vi "Get RD Data.vi"(8 "error in":errorcluster, 11 "tCRD in":refnum<class "tCRD.lvclass">) -> (0 "error out":errorcluster, 3 "tCRD out":refnum<class "tCRD.lvclass">)   [LabVIEW 2015, in "tCRD.lvclass"]
uses:
  tCRD.lvclass
  tCRD.lvclass/tCRD.ctl
  Reusable/Instrument/Instrument.lvclass/Instrument.ctl
  Reusable/CRDS/Main/CRDS.lvclass/CRDS.ctl
  Accessors/Read FPGA Ref.vi
  Accessors/Read RepRate.vi
  Accessors/Read SamplesPerRep.vi
  Reusable/Instrument/Write Restart Requested_.vi
  Reusable/CRDS/Main/Write Laser Data.vi
  <vilib>/Utility/error.llb/Error Cluster From Error Code.vi
  <vilib>/rvi/errors/niLvFpgaAdjustHostInterfaceError.vi
  tFPGA Ref.ctl
  <vilib>/rvi/interface/nirviMethod/nirviMethod.xnode
  FPGA Bitfiles/Handix_OpenPathCRD.lvbitx
  <vilib>/FPGAPlugInAG/sbRIO-9637/niLvFpga_ReadFifo_sbRIO-9637.vi
  <vilib>/rvi/errors/niLvFpgaMergeErrorWithErrorCode.vi
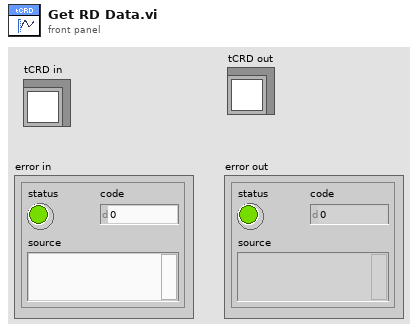
[diagram p1: front panel]
types:
  T1 = typedef "tCRD.lvclass/tFPGA Ref.ctl" = refnum<k20>
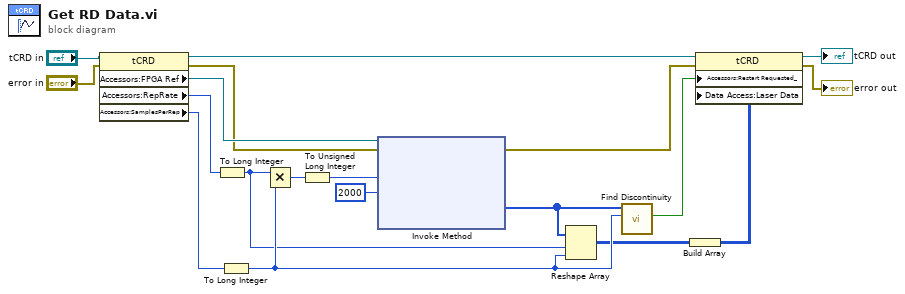
[diagram p0: block diagram]
diagram:
  n1 = property class="tCRD"(reference="tCRD in", error in="error in") -> (reference out=w1:refnum<class "tCRD.lvclass">, error out=w3:errorcluster, "Accessors:FPGA Ref"=w10:T1, "Accessors:RepRate"=w12:u16, "Accessors:SamplesPerRep"=w11:u16)
  n2 = To Long Integer(number=w12) -> (32bit integer=w15:i32)
  n3 = To Long Integer(number=w11) -> (32bit integer=w19:i32)
  n4 = Multiply(x=w15, y=w19) -> (x*y=w14:i32)
  n5 = To Unsigned Long Integer(number=w14) -> (unsigned 32bit integer=w16:u32)
  n6 = xnode "Invoke Method"("FPGA VI Reference In"=w10, "error in"=w3, "Number of Elements"=w16, "Timeout (ms)"=2000) -> ("error out"=w5:errorcluster, "Data"=w18:i16[])  [unwired: 2 out]
  n7 = Reshape Array(w18, w15, w19) -> (w2:i16[][])
  n8 = call "Find Discontinuity.vi"("Single Record"=w19, "Data"=w18) -> ("Discontinuity Detected"=w9:bool)  [unwired: 8 in, 1 out]
  n9 = Build Array(w2) -> (w8:i16[][][])
  n10 = property class="tCRD"(reference=w1, error in=w5, "Accessors:Restart Requested_"=w9, "Data Access:Laser Data"=w8) -> (reference out=→"tCRD out":refnum<class "tCRD.lvclass">, error out=→"error out":errorcluster)
